vi "put.vi"(8 "error in (no error)":errorcluster, 9 "pShape.lvclass":refnum<class "pShape.lvclass">, 10 "Key":string, 11 "BundledShapeCache in":refnum<class "BundledShapeCache.lvclass">) -> (0 "error out":errorcluster, 3 "BundledShapeCache out":refnum<class "BundledShapeCache.lvclass">)   [LabVIEW 2018, in "BundledShapeCache.lvclass"]
uses:
  BundledShapeCache.lvclass
  Shape Class/pShape.lvclass
  BundledShapeCache.lvclass/BundledShapeCache.ctl
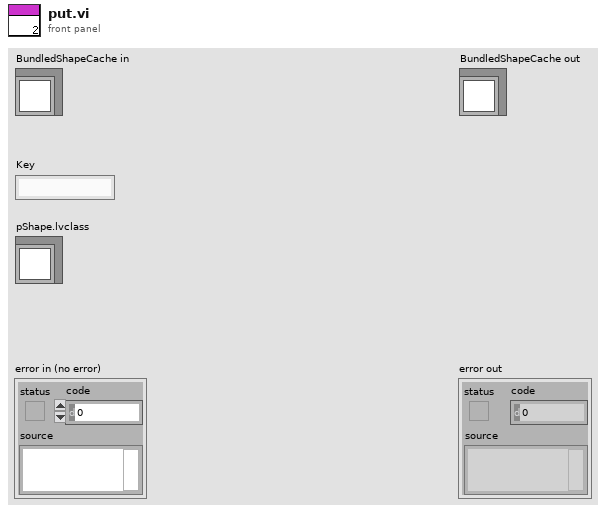
[diagram p1: front panel]
types:
  T1 = cluster{"String":string, "pShape.lvclass":refnum<class "pShape.lvclass">}[]
  T2 = cluster{"Key":string, "pShape.lvclass":refnum<class "pShape.lvclass">}
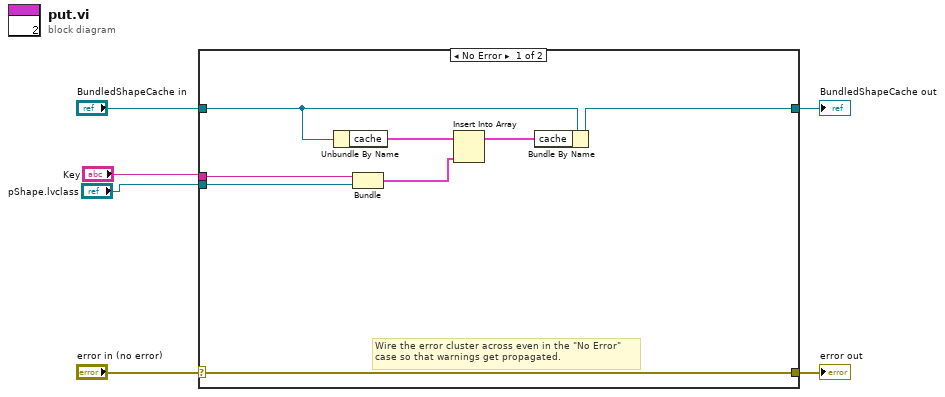
[diagram p0: block diagram]
diagram:
  n1 = case shown="No Error" "error in (no error)" {
    selector: "error in (no error)" -> [w14 w16]
    tunnel: [w14 w16] -> w5
    tunnel: [w10 w15] -> w3
    tunnel: "BundledShapeCache in" -> [w13 w15]
    tunnel: "Key" -> [w12 _]
    tunnel: "pShape.lvclass" -> [w11 _]
    frame No Error {
      # "Wire the error cluster across even in the \"No Error\"\ncase so that warnings get propagated."
      n2 = Unbundle By Name(w13) -> ("cache"=w9:T1)
      n3 = Bundle("Key"=w12, "pShape.lvclass"=w11) -> (w7:T2)  [unwired: 1 in]
      n4 = Insert Into Array(array=w9, new element=w7) -> (w8:T1)  [unwired: 1 in]
      n5 = Bundle By Name(cluster=w13, "cache"=w8) -> (w10:refnum<class "BundledShapeCache.lvclass">)
    }
    frame Error {
    }
  }
  "error out" <- w5
  "BundledShapeCache out" <- w3
